vi "CTRE_Phoenix_CANdle_TwinkleOffAnimation.vi"(0 "CTRE_CANdle_DeviceRef":T3, 1 "Twinkle Percent":T1 items=["100 Percent", "88 Percent", "76 Percent", "64 Percent", "42 Percent", "30 Percent", "18 Percent", "6 Percent"], 5 "Speed":dbl=1.0 min=0.0 max=1.0 step=0.0001, 7 "Num LEDs":i32=-1, 9 "LED Color":T2, 11 "error in":errorcluster) -> (4 "CTRE_CANdle_DeviceRef":T3, 15 "error out":errorcluster)   [LabVIEW 2020]
doc: "Animation that randomly turns on LEDs, until it reaches the maximum count and turns them all off\n\n<b>Speed</b> adjust the speed at which the animation runs. Valid values range from 0 to 1 where 1 is the fastest animation speed.\n\n<b>Num LEDs</b> defines the total number of LEDs to use for the animation.\n\n<b>LED Color</b> is the RGB(W) value of the color to illuminate.\n\n<b>Twinkle Percent</b> is what percent of the LEDs can be on at any given time."
uses:
  <vilib>/Rock Robotics/WPI/ThirdParty/Phoenix-LabVIEW/CANdle/Controls/CTRE_Phoenix_CANdle_DeviceRef.ctl
  <vilib>/Rock Robotics/WPI/ThirdParty/Phoenix-LabVIEW/CANdle/Controls/CTRE_Phoenix_CANdle_LEDColor.ctl
  <vilib>/Rock Robotics/WPI/ThirdParty/Phoenix-LabVIEW/CANdle/Controls/CTRE_Phoenix_CANdle_AnimationTwinklePercent.ctl
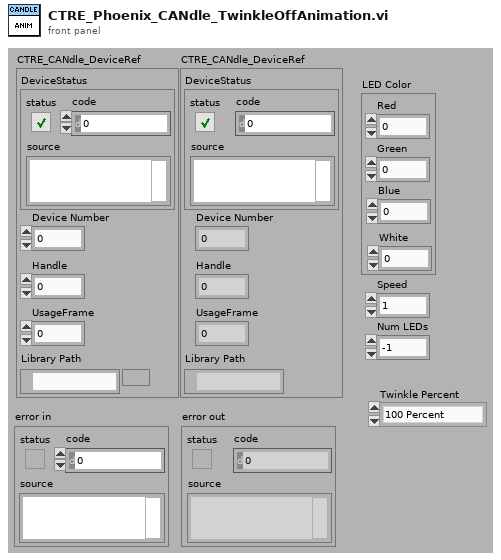
[diagram p1: front panel]
types:
  T1 = typedef "CTRE_Phoenix_CANdle_AnimationTwinklePercent.ctl" = u16
  T2 = typedef "CTRE_Phoenix_CANdle_LEDColor.ctl" = cluster{"Red":u8, "Green":u8, "Blue":u8, "White":u8}
  T3 = typedef "CTRE_Phoenix_CANdle_DeviceRef.ctl" = cluster{"DeviceStatus":errorcluster, "Device Number":u8, "Handle":u64, "UsageFrame":u32, "Library Path":path}
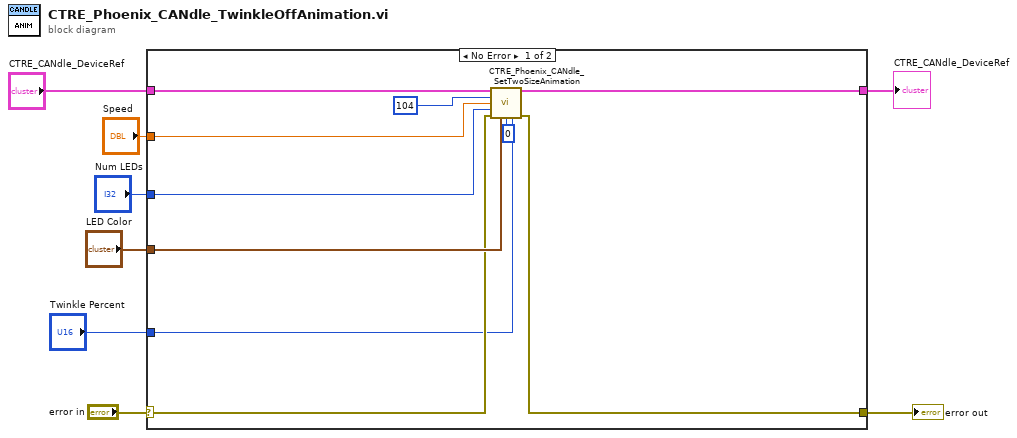
[diagram p0: block diagram]
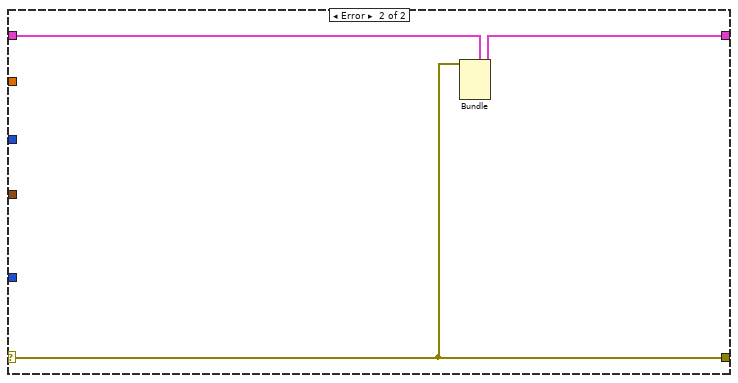
[diagram p2: hidden frame]
diagram:
  n1 = case shown="No Error" "error in" {
    selector: "error in" -> [w12 w20]
    tunnel: "CTRE_CANdle_DeviceRef" -> [w18 w21]
    tunnel: [w11 w20] -> w8
    tunnel: [w17 w19] -> w5
    tunnel: "LED Color" -> [w16 _]
    tunnel: "Speed" -> [w14 _]
    tunnel: "Num LEDs" -> [w13 _]
    tunnel: "Twinkle Percent" -> [w9 _]
    frame No Error {
      n2 = call <vilib>:"CTRE_Phoenix_CANdle_SetTwoSizeAnimation.vi"("CTRE_CANdle_DeviceRef"=w18, "idx"=104, "speed"=w14, "numLED"=w13, "error in"=w12, "LED Color"=w16, "direction"=0, "size"=w9) -> ("CTRE_CANdle_DeviceRef"=w17:T3, "error out"=w11:errorcluster)  [unwired: 6 in]
    }
    frame Error {
      n3 = Bundle(cluster=w21, "DeviceStatus"=w20) -> (w19:T3)  [unwired: 4 in]
    }
  }
  "error out" <- w8
  "CTRE_CANdle_DeviceRef" <- w5
